vi "Array Manipulation 2.vi"() -> ()   [LabVIEW 2022 SP3]
uses:
  <vilib>/measure/NI_MABase.lvlib
panel:
  in  "Tab Control":T1(tab)
  out "Array":dbl[](array[numeric])
  out "Concatenated Data":dbl[](graph)
  out "Add/Subtract Channel":dbl[](graph)
  in  "Subtract":bool
  out "Add/Subtract Array Data":dbl[](array[numeric])
  in  "Enum":enum16{"Channel 0", "Channel 1"}(ring)
  out "Single Channel of Data Array":dbl[](array[numeric])
  out "Single Channel of Data":dbl[](graph)
  in  "Offset":dbl(slide) scale=0.0..10.0
  out "Waveform Data":waveform(dbl)[](graph)
  out "Waveform Data 2":dbl[][](graph)
  in  "Offset 2":dbl(slide) scale=0.0..10.0
  out "Waveform Data3":dbl[][](graph)
  out "Subset Data Array":dbl[][](array[numeric])
  in  "Length":dbl(slide)=1000.0 scale=0.0..1000.0
  in  "Start Value":dbl(slide) scale=0.0..1000.0
  out "Waveform Data3 2":dbl[][](graph)
  in  "Stop":bool
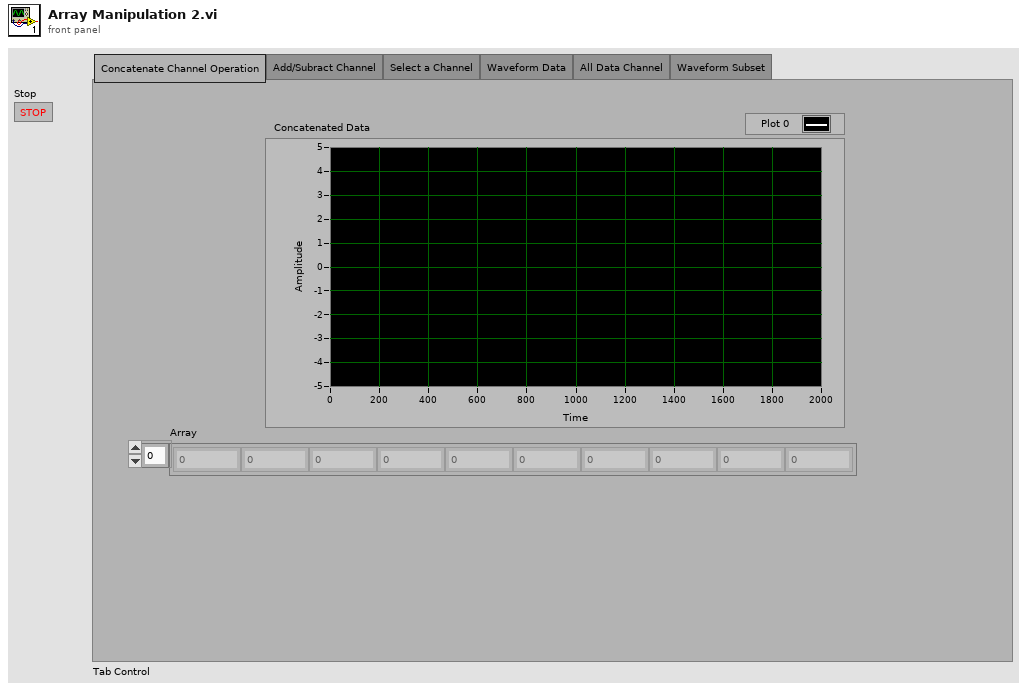
[diagram p1: front panel]
types:
  T1 = enum32{"Concatenate Channel Operation", "Add/Subract Channel", "Select a Channel", "Waveform Data", "All Data Channel", "Waveform Subset"}
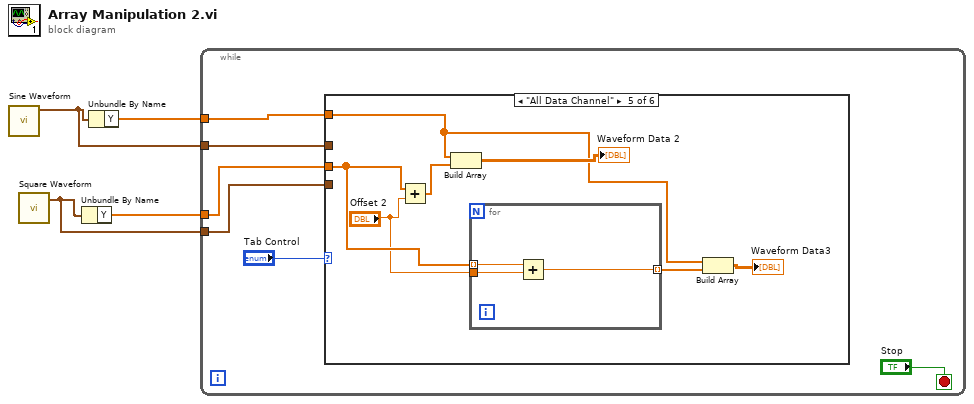
[diagram p0: block diagram]
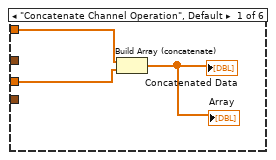
[diagram p2: hidden frame]
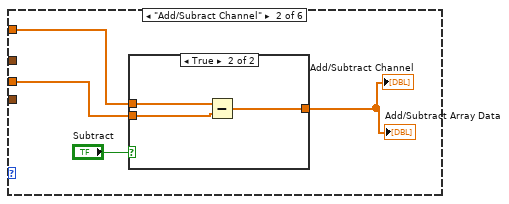
[diagram p3: hidden frame]
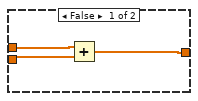
[diagram p4: hidden frame]
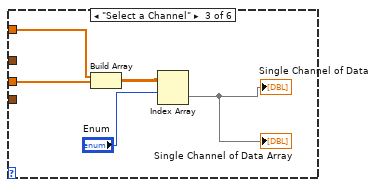
[diagram p5: hidden frame]
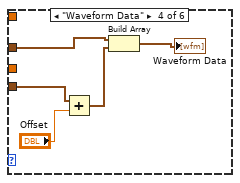
[diagram p6: hidden frame]
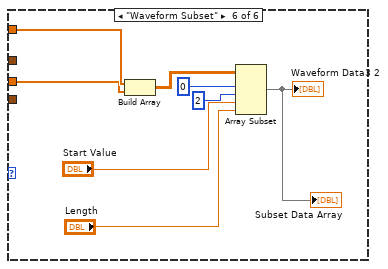
[diagram p7: hidden frame]
diagram:
  n1 = call <vilib>:"Sine Waveform.vi"() -> ("signal out"=w3:waveform(dbl))  [unwired: 10 in, 1 out]
  n2 = call <vilib>:"Square Waveform.vi"() -> ("signal out"=w1:waveform(dbl))  [unwired: 10 in, 1 out]
  n3 = Unbundle By Name(w1) -> ("Y"=w2:dbl[])
  n4 = Unbundle By Name(w3) -> ("Y"=w4:dbl[])
  n5 = while {
    tunnel: w4 -> [w9]
    tunnel: w3 -> [w8]
    tunnel: w2 -> [w7]
    tunnel: w1 -> [w6]
    stop <- "Stop" stop-if-true
    n6 = case shown="\"All Data Channel\"" "Tab Control" {
      tunnel: w9 -> [w13 w16 w28 _ w35 w51]
      tunnel: w8 -> [_ _ _ w29 _ _]
      tunnel: w7 -> [w12 w15 w27 _ w38 w50]
      tunnel: w6 -> [_ _ _ w33 _ _]
      frame "Concatenate Channel Operation", Default {
        n7 = Build Array (concatenate) "Build Array"(w13, w12) -> (→"Concatenated Data" →"Array":dbl[])
      }
      frame "Add/Subract Channel" {
        n8 = case shown="True" "Subtract" {
          tunnel: w16 -> [w20 w23]
          tunnel: w15 -> [w19 w22]
          tunnel: [w18 w21] -> w14
          frame False {
            n9 = Add(x=w20, y=w19) -> (x+y=w18:dbl[])
          }
          frame True {
            n10 = Subtract(x=w23, y=w22) -> (x-y=w21:dbl[])
          }
        }
        "Add/Subtract Channel" <- w14
        "Add/Subtract Array Data" <- w14
      }
      frame "Select a Channel" {
        n11 = Build Array "Build Array"(w28, w27) -> (w26:dbl[][])
        n12 = Index Array(array=w26, index (row)="Enum") -> (element=→"Single Channel of Data" →"Single Channel of Data Array":dbl[])  [unwired: 1 in]
      }
      frame "Waveform Data" {
        n13 = Add(x=w33, y="Offset") -> (x+y=w30:waveform(dbl))
        n14 = Build Array(w29, w30) -> (→"Waveform Data":waveform(dbl)[])
      }
      frame "All Data Channel" {
        n15 = Add(x=w38, y="Offset 2") -> (x+y=w40:dbl[])
        n16 = Build Array(w35, w40) -> (→"Waveform Data 2":dbl[][])
        n17 = for {
          tunnel: w38 -> [w43] mode=indexing
          tunnel: "Offset 2" -> [w42]
          tunnel: [w41] -> w36 mode=indexing
          n18 = Add(x=w43, y=w42) -> (x+y=w41:dbl)
        }
        n19 = Build Array(w35, w36) -> (→"Waveform Data3":dbl[][])
      }
      frame "Waveform Subset" {
        n20 = Build Array(w51, w50) -> (w49:dbl[][])
        n21 = Array Subset(array=w49, index (row)=0 ("index"), length (row)=2 ("length"), index (col)="Start Value", length (col)="Length") -> (→"Waveform Data3 2" →"Subset Data Array":dbl[][])
      }
    }
  }
